vi "Read ByteArray.vi"(8 "error in":errorcluster, 9 "count (-1: all)":i32=-1, 11 "Buffer":refnum<data-value>) -> (0 "error out":errorcluster, 2 "bytes":u8[](array[numeric]) format="%02x", 3 "Buffer":refnum<data-value>)   [LabVIEW 2013, in "CircularBuffer.lvlib" / "ByteFIFO.lvclass"]
doc: "This VI returns data from the ring buffer starting from the oldest data and ending with the newest.\n\nThe data is duplicated at the output so this VI allocates new place in the memory for the output."
uses:
  ByteFIFO.lvclass
  VariantBuffer/VariantBuffer.lvclass
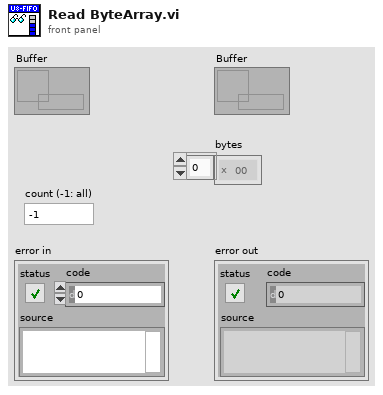
[diagram p1: front panel]
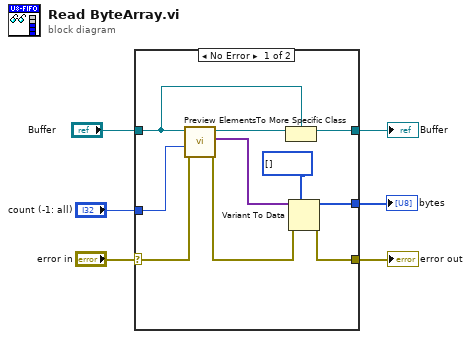
[diagram p0: block diagram]
diagram:
  n1 = case shown="No Error" "error in" {
    selector: "error in" -> [w14 w17]
    tunnel: "Buffer" -> [w7 w18]
    tunnel: [w8 w18] -> w5
    tunnel: [w9 w17] -> w3
    tunnel: [w12 _] -> w1
    tunnel: "count (-1: all)" -> [w15 _]
    frame No Error {
      n2 = call "Preview Elements.vi"("error in"=w14, "count (-1: all)"=w15, "ByteBuffer in"=w7) -> ("error out"=w10:errorcluster, "elements"=w13:variant[], "ByteBuffer"=w16:refnum<data-value>)  [unwired: 6 in]
      n3 = To More Specific Class(target class=w7, reference=w16) -> (specific class reference=w8:refnum<data-value>)  [unwired: 1 in, 1 out]
      n4 = Variant To Data(error in=w10, type=u8[] [] ("bytes"), Variant=w13) -> (data=w12:u8[], error out=w9:errorcluster)
    }
    frame Error {
    }
  }
  "error out" <- w3
  "Buffer" <- w5
  "bytes" <- w1
